vi "Variable@GetPointString__Parameter.vi"(1 "ParamterIn":string) -> (0 "ParamterOut":string)   [LabVIEW 2020]
panel:
  in  "Point":string(combo)
  in  "Section":string(combo)
  in  "Variable":string(combo)
  in  "Confirm":bool
  # "Variable@GetPointString $Variable,$Point(,Section)"
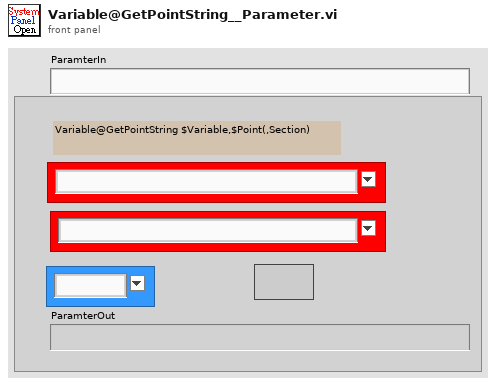
[diagram p1: front panel]
types:
  T1 = enum16{"Get", "UpdatePointS", "Init", "UpdateIndex", "GetCurrent&Index+1", "GetWithIndex", "ChkLast", "GetCurrent"}
  T2 = enum16{"Get", "Init", "Set", "Delete", "GetElement", "Inc", "Dec"}
  T3 = enum16{"Get", "Init", "Set", "Delete", "GetElement", "Inc", "Dec", "ReName"}
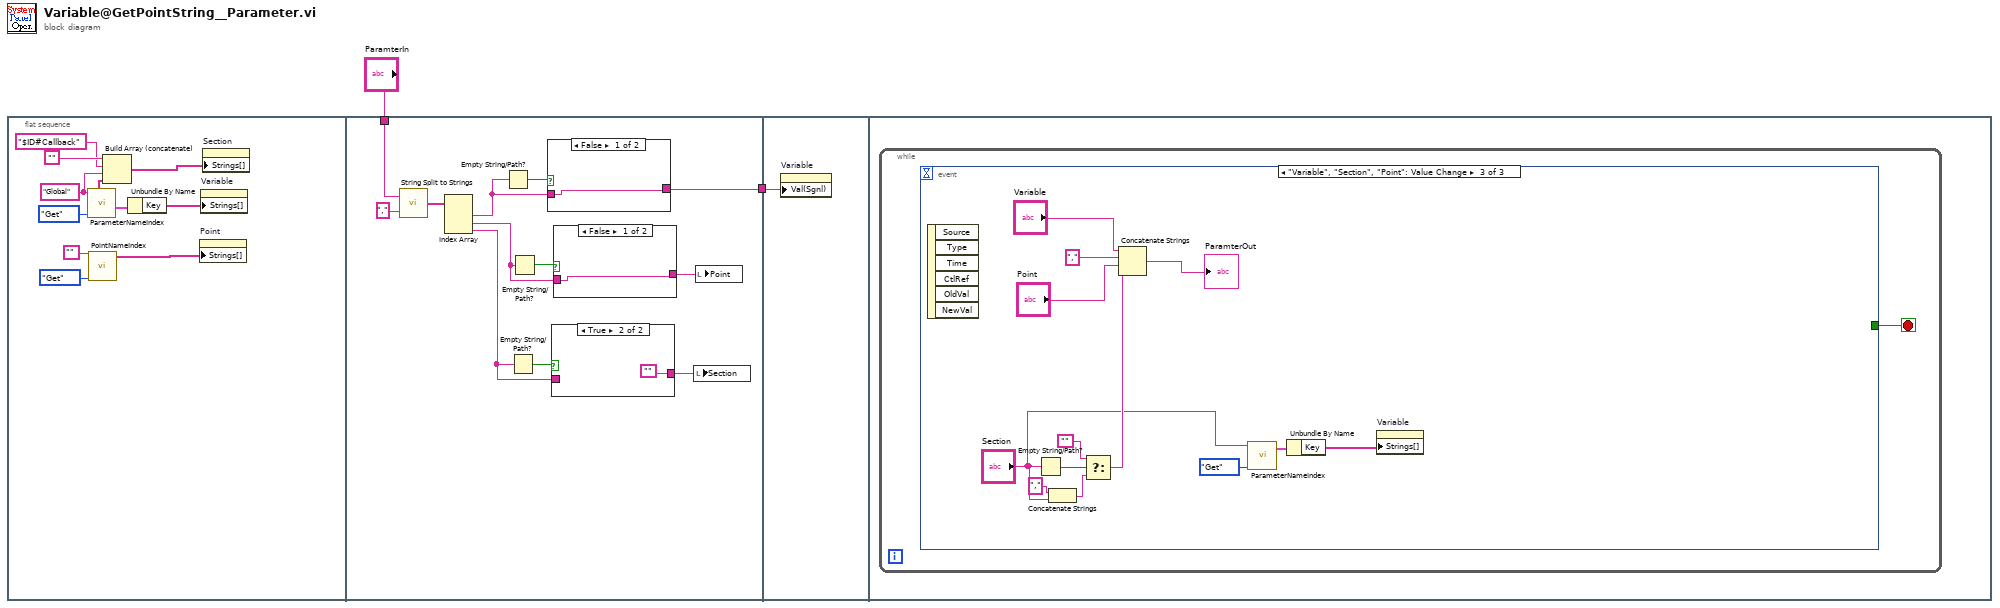
[diagram p0: block diagram]
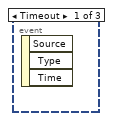
[diagram p5: hidden frame]
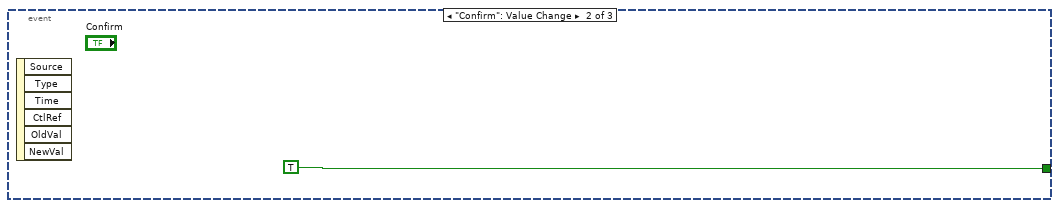
[diagram p6: hidden frame]
diagram:
  n1 = flat-sequence {
    tunnel: "ParamterIn" -> [w21]
    tunnel: [w23] -> w1
    tunnel: w1 -> [w32]
    frame #0 {
      w5 = "Global" ("VariableSection")
      n2 = call "ParameterNameIndex.vi"("OP"=T2."Get", "VariableSection"=w5) -> ("GlobalKeyValue"=w12:cluster{"Key":string[], "Value":string[]}, "SectionList"=w6:string[])  [unwired: 3 in, 5 out]
      n3 = call "PointNameIndex.vi"("OP"=T1."Get", "PointName"="") -> ("PointNameList"=w8:string[])  [unwired: 4 in, 5 out]
      n4 = Build Array (concatenate)("", "$ID#Callback" ("VariableSection"), w5, w6) -> (w4:string[])
      n5 = Unbundle By Name(w12) -> ("Key"=w11:string[])
      n6 = property on="Point" class="CmbBox"("Strings[]"=w8) -> ()  [unwired: 2 in, 2 out]
      n7 = property on="Variable" class="CmbBox"("Strings[]"=w11) -> ()  [unwired: 2 in, 2 out]
      n8 = property on="Section" class="CmbBox"("Strings[]"=w4) -> ()  [unwired: 2 in, 2 out]
    }
    frame #1 {
      n9 = call "String Split to Strings.vi"("search string/char (-)"=",", "String"=w21) -> ("Array"=w19:string[])
      n10 = Index Array(array=w19) -> (element #1=w18:string, element #2=w15:string, element #3=w17:string)  [unwired: 3 in]
      n11 = Empty String/Path?(string/path=w18) -> (empty?=w25:bool)
      n12 = Empty String/Path?(string/path=w17) -> (empty?=w24:bool)
      n13 = Empty String/Path?(string/path=w15) -> (empty?=w16:bool)
      n14 = case shown="False" w25 {
        tunnel: w18 -> [w30 w31]
        tunnel: [w30 w31] -> w23
        frame False {
        }
        frame True {
        }
      }
      n15 = case shown="True" w24 {
        tunnel: w17 -> [w28 _]
        tunnel: [w28 ""] -> w22
        frame False {
        }
        frame True {
        }
      }
      n16 = case shown="False" w16 {
        tunnel: w15 -> [w26 w27]
        tunnel: [w26 w27] -> w14
        frame False {
        }
        frame True {
        }
      }
      n17 = local write "Section"(w22) -> ()
      n18 = local write "Point"(w14) -> ()
    }
    frame #2 {
      n19 = property on="Variable" class="CmbBox"("Val(Sgnl)"=w32) -> ()  [unwired: 2 in, 2 out]
    }
    frame #3 {
      n20 = while {
        stop <- w33 stop-if-true
        n21 = event shown="[2] \"Variable\", \"Section\", \"Point\": Value Change" {
          selector: _ -> [_ _ _]
          dyn-events: _ -> [_ _ _]
          timeout: _ -> [_ _ _]
          tunnel: [_ TRUE _] -> w33
          event Timeout {
            n22 = event-data() -> ()  [unwired: 1 in, 3 out]
          }
          event "Confirm": Value Change {
            n23 = event-data() -> ()  [unwired: 1 in, 6 out]
          }
          event "Variable", "Section", "Point": Value Change {
            n24 = event-data() -> ()  [unwired: 1 in, 6 out]
            n25 = Empty String/Path?(string/path="Section") -> (empty?=w45:bool)
            n26 = Concatenate Strings("," ("string"), "Section") -> (w43:string)
            n27 = Select(t="", s=w45, f=w43) -> (s? t:f=w39:string)
            n28 = Concatenate Strings("Variable", "," ("string"), "Point", w39) -> (→"ParamterOut":string)
            n29 = call "ParameterNameIndex.vi"("OP"=T3."Get", "VariableSection"="Section") -> ("SectionKeyValue"=w36:cluster{"Key":string[], "Value":string[]})  [unwired: 3 in, 6 out]
            n30 = Unbundle By Name(w36) -> ("Key"=w38:string[])
            n31 = property on="Variable" class="CmbBox"("Strings[]"=w38) -> ()  [unwired: 2 in, 2 out]
          }
        }
      }
    }
  }
